vi "Continuous IQ ACquisition.vi"() -> ()   [LabVIEW 2022 SP3]
uses:
  <instrlib>/niUSRP/niUSRP Fetch Rx Data (CDB Cluster).vi
  <vilib>/addons/Modulation/niAMT.lvlib
panel:
  out "Real Graph 2":cluster{"t0":dbl, "dt":dbl, "Y":dbl[]}(graph)
  out "Waveform Graph":cluster{"t0":dbl, "dt":dbl, "Y":dbl[]}(graph)
  in  "number of samples":i64=100000
  out "coerced gain":dbl format="%#_6f"
  out "coerced carrier frequency":dbl=100000.0 format="%#_6p"
  out "coerced IQ rate":dbl=100000.0 format="%#_6p"
  in  "active antenna 2":string
  in  "gain (dB)":dbl
  in  "?":bool
  in  "frequency (Hz)":dbl
  in  "IQ rate (S/s)":dbl
  in  "USRP IP Address":refnum<k15>
  out "error out":errorcluster
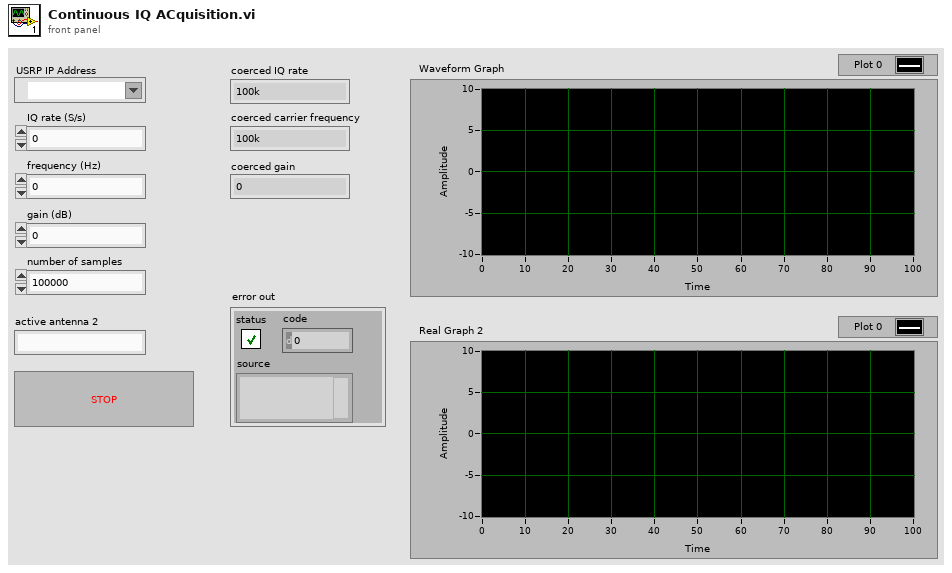
[diagram p1: front panel]
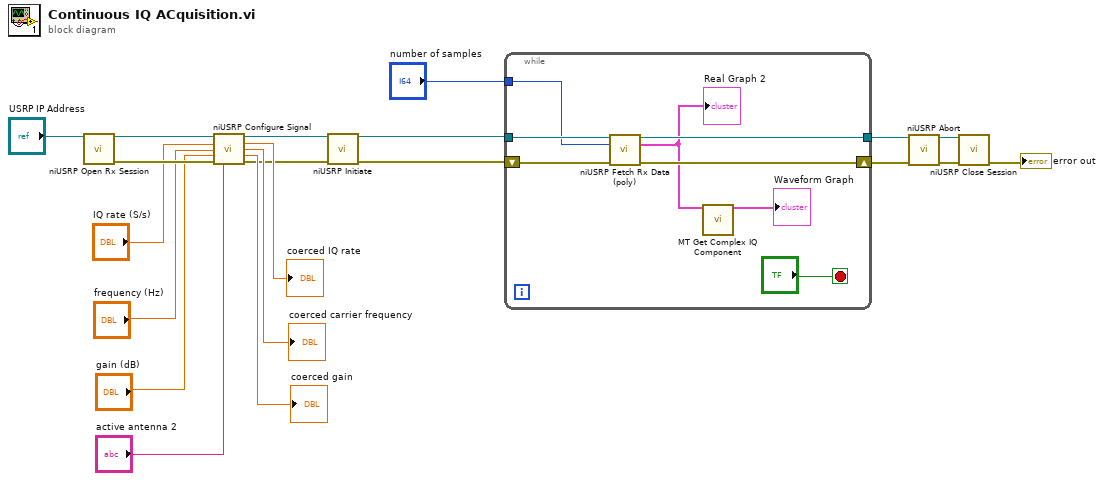
[diagram p0: block diagram]
diagram:
  n1 = call <instrlib>:"niUSRP Open Rx Session.vi"("device names"="USRP IP Address") -> ("session handle out"=w18:refnum<k15>, "error out"=w20:errorcluster)  [unwired: 13 in]
  n2 = call <instrlib>:"niUSRP Configure Signal.vi"("session handle"=w18, "IQ rate"="IQ rate (S/s)", "carrier frequency"="frequency (Hz)", "gain"="gain (dB)", "error in (no error)"=w20, "active antenna"="active antenna 2") -> ("session handle out"=w8:refnum<k15>, "coerced IQ rate"=→"coerced IQ rate":dbl, "coerced carrier frequency"=→"coerced carrier frequency":dbl, "coerced gain"=→"coerced gain":dbl, "error out"=w7:errorcluster)  [unwired: 5 in]
  n3 = call <instrlib>:"niUSRP Initiate.vi"("session handle"=w8, "error in (no error)"=w7) -> ("session handle out"=w6:refnum<k15>, "error out"=w5:errorcluster)  [unwired: 12 in]
  n4 = while {
    tunnel: w6 -> [w26]
    tunnel: [w25] -> w17
    tunnel: "number of samples" -> [w23]
    shift-right: [w27] -> w19
    shift-left: w5 -> [w28]
    stop <- "?" stop-if-true
    n5 = call-poly <instrlib>:"niUSRP Fetch Rx Data (poly).vi"("session handle"=w26, "number of samples"=w23, "error in (no error)"=w28) -> ("session handle out"=w25:refnum<k15>, "data"=w22:cluster{"t0":dbl, "dt":dbl, "Y":cdb[]}, "error out"=w27:errorcluster)  [unwired: 9 in, 1 out]
    "Real Graph 2" <- w22
    n6 = call <vilib>:"MT Get Complex IQ Component.vi"("IQ data (complex) in"=w22) -> ("IQ data (complex) out"=→"Waveform Graph":cluster{"t0":dbl, "dt":dbl, "Y":cdb[]})  [unwired: 12 in, 2 out]
  }
  n7 = call <instrlib>:"niUSRP Abort.vi"("session handle"=w17, "error in (no error)"=w19) -> ("session handle out"=w3:refnum<k15>, "error out"=w2:errorcluster)  [unwired: 12 in]
  n8 = call <instrlib>:"niUSRP Close Session.vi"("session handle"=w3, "error in (no error)"=w2) -> ("error out"=→"error out":errorcluster)  [unwired: 13 in]
